vi "IMS Stepper Read Position.vi"(2 "error in (no error)":errorcluster, 3 "Motor Number":u32=1 min=1 max=255 step=1, 4 "Instrument Address":refnum<visa-resource-name>) -> (0 "error out":errorcluster, 1 "Response":dbl format="%.4f")   [LabVIEW 2018]
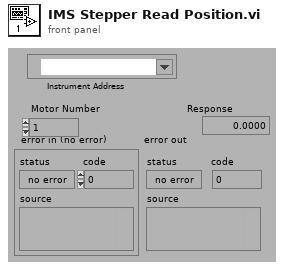
[diagram p1: front panel]
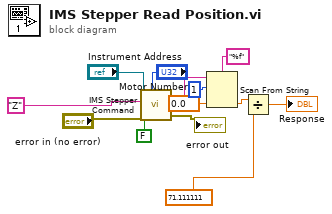
[diagram p0: block diagram]
diagram:
  n1 = call "IMS Stepper Command.vi"("Instrument Address"="Instrument Address", "Motor Number"="Motor Number", "Command"="Z", "Mode"=FALSE, "error in (no error)"="error in (no error)") -> ("Response"=w6:string, "error out"=→"error out":errorcluster)  [unwired: 1 in, 1 out]
  n2 = Scan From String(format string="%f", input string=w6, initial scan location=u32 1, default 1=0.0 ("default value 1")) -> (output 1=w8:dbl)  [unwired: 1 in, 3 out]
  n3 = Divide(x=w8, y=71.111111) -> (x/y=→"Response":dbl)
